vi "TLB Native Dynamic Events ver 0.07a.vi"() -> ()   [LabVIEW 2018]
uses:
  Labview Training Phase 2/Enum Controls/States for Action Engine.ctl
  Type def/TLB event states.ctl
  Type def/TLB MHL States.ctl
  <vilib>/Studica/Studica Toolkit/Background/I2C Channel.ctl
  <vilib>/Studica/Studica Toolkit/NavX/NavX.lvlib
  <vilib>/myRIO/Common/Instrument Driver Framework/myRIO v1.0/AI/typedefs/AI Channels Enum.ctl
  <vilib>/myRIO/Common/Instrument Driver Framework/myRIO v1.0/AI/typedefs/AI Channels List.ctl
  Type def/Type def.ctl
  Type def/Motor Control Cluster.ctl
  <vilib>/Studica/Studica Blackhawk/Blackhawk.lvlib
  <vilib>/userdefined/High Color/IMAQdx.ctl
  Underlying VI's/Webcam FGV Low level ver/State control.ctl
  <vilib>/Studica/Studica Toolkit/Background/Mxp Selection.ctl
  <vilib>/ptbypt/NI_PtbyPt.lvlib
  <vilib>/Studica/Studica Toolkit/Background/DIO Channel.ctl
  <vilib>/addons/control/pid/NI_PID_pid.lvlib
  <vilib>/addons/control/pid/pid.llb/PID (DBL).vi
  <vilib>/NI_Real-Time Target Support.lvlib
  <vilib>/Utility/RT CPU Load.ctl
panel:
  out "Load":errorcluster
  out "CPU loads":T1[](array[typedef]) {"ISR (%)" format="%#.2f"; "Idle (%)" format="%#.2f"; "Background (%)" format="%#.2f"; "Normal (%)" format="%#.2f"; "Above Normal (%)" format="%#.2f"; "High (%)" format="%#.2g"; "Timed Structures (%)" format="%#.2g"; "Time Critical (%)" format="%#.2g"; "Total (%)" format="%#.2g"}
  out "Waveform Chart":dbl(graph)
  in  "STOP":bool
  out "DIO 0":bool
  out "DIO 1":bool
  out "Limit Switch Array":bool[](array[boolean])
  out "Speed and distance cluster":T2
  out "error out":errorcluster
  out "Blackhawk loop":i32
  out "NavX Loop":i32
  out "Sensor Loop":i32
  out "User event loop":i32
  out "Event handling loop":i32
  out "Main Loop":i32
  out "Status loop":i32
  out "L/R average":fxp<+,64,64>
  out "Right Ultrasonic":fxp<+,64,16>
  out "Left Ultrasonic":fxp<+,64,16>
  out "Object detection count":T3
  out "Camera error":errorcluster
  out "Right IR Sensor":dbl
  out "Left IR Sensor":dbl
  in  "Servo Angle":u8(slide) scale=0.0..180.0
  in  "On/Off":bool
  out "Blackhawk error":errorcluster
  out "element":T4
  out "Action Queue Items":i32
  out "State Logic Queue Items":i32
  out "Action Queues items":string[](array[string])=["Hardware reset", "Software reset", ""]
  out "State logic":T5=enum."Task 2"
  out "Action State":string
  in  "Tasks Selector":string(combo)="Drive straight"
  out "Yaw":dbl
  out "NavX Info Out":T7
  out "LinearAcceleration":T8
  out "Displacement":T9
  out "YRPHfH":T10
  out "Object detected":bool
  in  "NavX Zero Yaw":bool
  # "Camera Status Loop"
  # "TLB FRAMEWORK STATUS"
  # "Test Programme written by Calvin Loke    Dated: 28 Aug 2019\nTest Programme revised by Dr Alex See   Dated 30 Aug 2019\n\nProgramme version:   TLB Native Dynamic Events ver 0.04b.vi"
  # "Sequence of Actions"
  # "Continuous (Repeated)"
  # "Motor Control Loop"
  # "Sensor data"
  # "Blackhawk status"
  # "System Health Status Update"
  # "NAVX Control Loop"
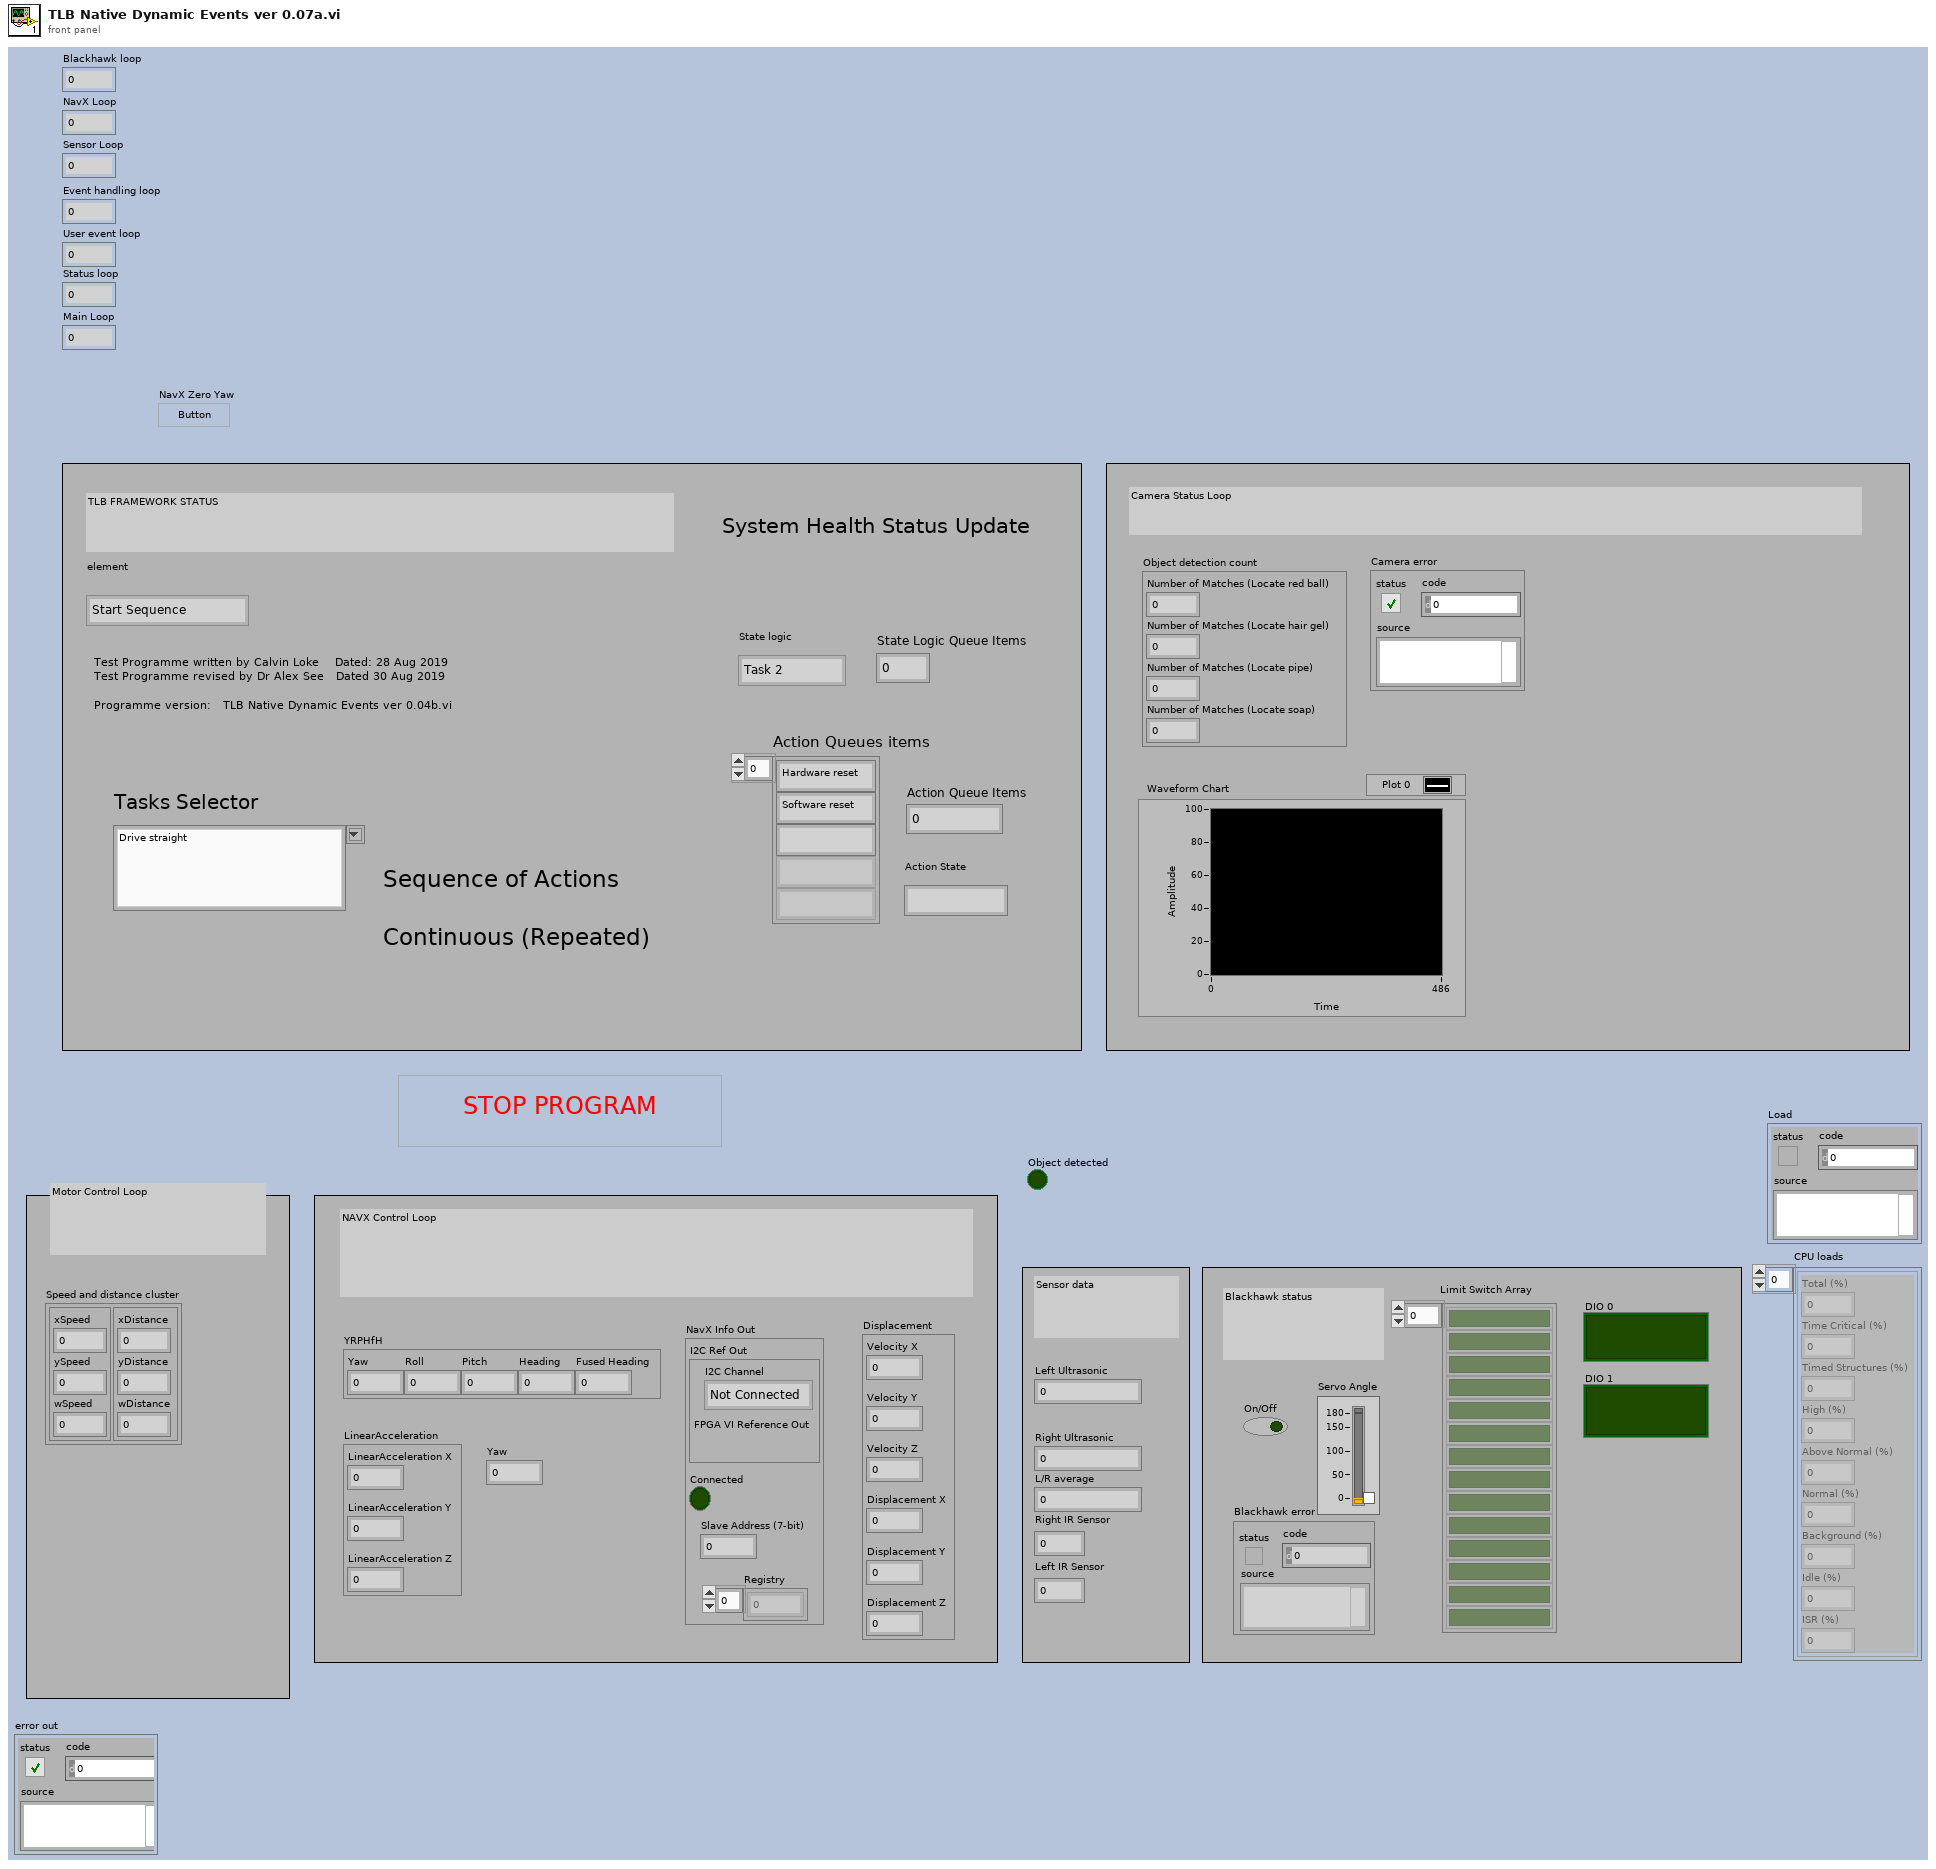
[diagram p1: front panel]
types:
  T1 = typedef "NI_Real-Time Target Support.lvlib/RT CPU Load.ctl" = cluster{"Total (%)":dbl, "Time Critical (%)":dbl, "Timed Structures (%)":dbl, "High (%)":dbl, "Above Normal (%)":dbl, "Normal (%)":dbl, "Background (%)":dbl, "Idle (%)":dbl, "ISR (%)":dbl}
  T2 = cluster{cluster{"xSpeed":dbl, "ySpeed":dbl, "wSpeed":dbl}, cluster{"xDistance":dbl, "yDistance":dbl, "wDistance":dbl}}
  T3 = cluster{"Number of Matches (Locate red ball)":i32, "Number of Matches (Locate hair gel)":i32, "Number of Matches (Locate pipe)":i32, "Number of Matches (Locate soap)":i32}
  T4 = typedef "TLB event states.ctl" = enum16{"Start Sequence", "Exit", "Start Task 1", "Start Task 2", "Start Task 3", "Start Task 4", "Camera vision", "Wall follow mode", "Idle", "Start Drive Straight"}
  T5 = typedef "TLB MHL States.ctl" = enum16{"None", "Startup", "Idle", "Processing", "Shutdown", "Reset", "Task 1", "Task 2", "Task 3", "Task 4", "Task 4a", "Task 4b", "Task 4c", "Task 4d", "Task 4e", "Task 4f", "Task 4g", "Task 4h", "Acquire image", "Wall follow mode", "Autodrive", "Autodrive a"}
  T6 = typedef "I2C Channel.ctl" = enum16{"Not Connected", "A", "B"}
  T7 = cluster{"I2C Ref Out":cluster{"I2C Channel":T6, "FPGA VI Reference Out":refnum<k20>}, "Connected":bool, "Slave Address (7-bit)":u8, "Registry":u8[]}
  T8 = cluster{"LinearAcceleration X":dbl, "LinearAcceleration Y":dbl, "LinearAcceleration Z":dbl}
  T9 = cluster{"Velocity X":dbl, "Velocity Y":dbl, "Velocity Z":dbl, "Displacement X":dbl, "Displacement Y":dbl, "Displacement Z":dbl}
  T10 = cluster{"Yaw":dbl, "Roll":dbl, "Pitch":dbl, "Heading":dbl, "Fused Heading":dbl}
  T11 = typedef "States for Action Engine.ctl" = enum16{"Initialize", "Write", "Read"}
  T12 = typedef "DIO Channel.ctl" = enum16{"Not Connected", "A/DIO1", "A/DIO2", "A/DIO3", "A/DIO4", "A/DIO5", "A/DIO6", "A/DIO7", "A/DIO13", "B/DIO1", "B/DIO2", "B/DIO3", "B/DIO4", "B/DIO5", "B/DIO6", "B/DIO7", "B/DIO13", "C/DIO0", "C/DIO1", "C/DIO2", "C/DIO3", "C/DIO4", "C/DIO5", "C/DIO6", "C/DIO7"}
  T13 = typedef "Motor Control Cluster.ctl" = cluster{"Vx":dbl, "Vy":dbl, "Vw":dbl}
  T14 = typedef "Type def.ctl" = cluster{"Front Ultrasonic Obstruct":bool, "Left Ultrasonic Obstruct":bool, "Right Ultrasonic Obstruct ":bool}
  T15 = typedef "Mxp Selection.ctl" = enum16{"MXP A", "MXP B"}
  T16 = typedef "TLB MHL States.ctl" = enum16{"None", "Startup", "Idle", "Processing", "Shutdown", "Reset", "Task 1", "Task 2", "Task 3", "Task 4", "Task 4a", "Task 4b", "Task 4c", "Task 4d", "Task 4e", "Task 4f", "Task 4g", "Task 4h", "Acquire image", "Wall follow mode", "Drive Straight"}
  T17 = cluster{"proportional gain (Kc)":dbl, "integral time (Ti, min)":dbl, "derivative time (Td, min)":dbl}
  T18 = typedef "State control.ctl" = enum16{"Initialise", "Start camera", "Continuous Acquisition ", "Stop camera", "Dispose all"}
  T19 = typedef "IMAQdx.ctl" = refnum<k21>
  T20 = cluster{"xTargetSpeed":dbl, "yTargetSpeed":dbl, "wTargetSpeed":dbl}
  T21 = cluster{"DIO Channel":T12, "FPGA VI Reference Out":refnum<k20>}
  T22 = typedef "IMAQ Image.ctl" = refnum<image>
  T23 = cluster{"xDistance":dbl, "yDistance":dbl, "wDistance":dbl}
  T24 = typedef "AI Channels List.ctl" = T25[]
  T25 = typedef "AI Channels Enum.ctl" = enum16{"Not Connected", "AudioIn/Left", "AudioIn/Right", "C/AI0", "C/AI1", "A/AI0", "A/AI1", "A/AI2", "A/AI3", "A/AI4", "A/AI5", "A/AI6", "A/AI7", "B/AI0", "B/AI1", "B/AI2", "B/AI3", "B/AI4", "B/AI5", "B/AI6", "B/AI7", "AI/AI0", "AI/AI1", "AI/AI2", "AI/AI3", "A/AI0 (DIFF)", "A/AI1 (DIFF)", "A/AI2 (DIFF)", "A/AI3 (DIFF)", "B/AI0 (DIFF)", "B/AI1 (DIFF)", "B/AI2 (DIFF)", "B/AI3 (DIFF)"}
  T26 = cluster{"I2C Channel":T6, "FPGA VI Reference Out":refnum<k20>}
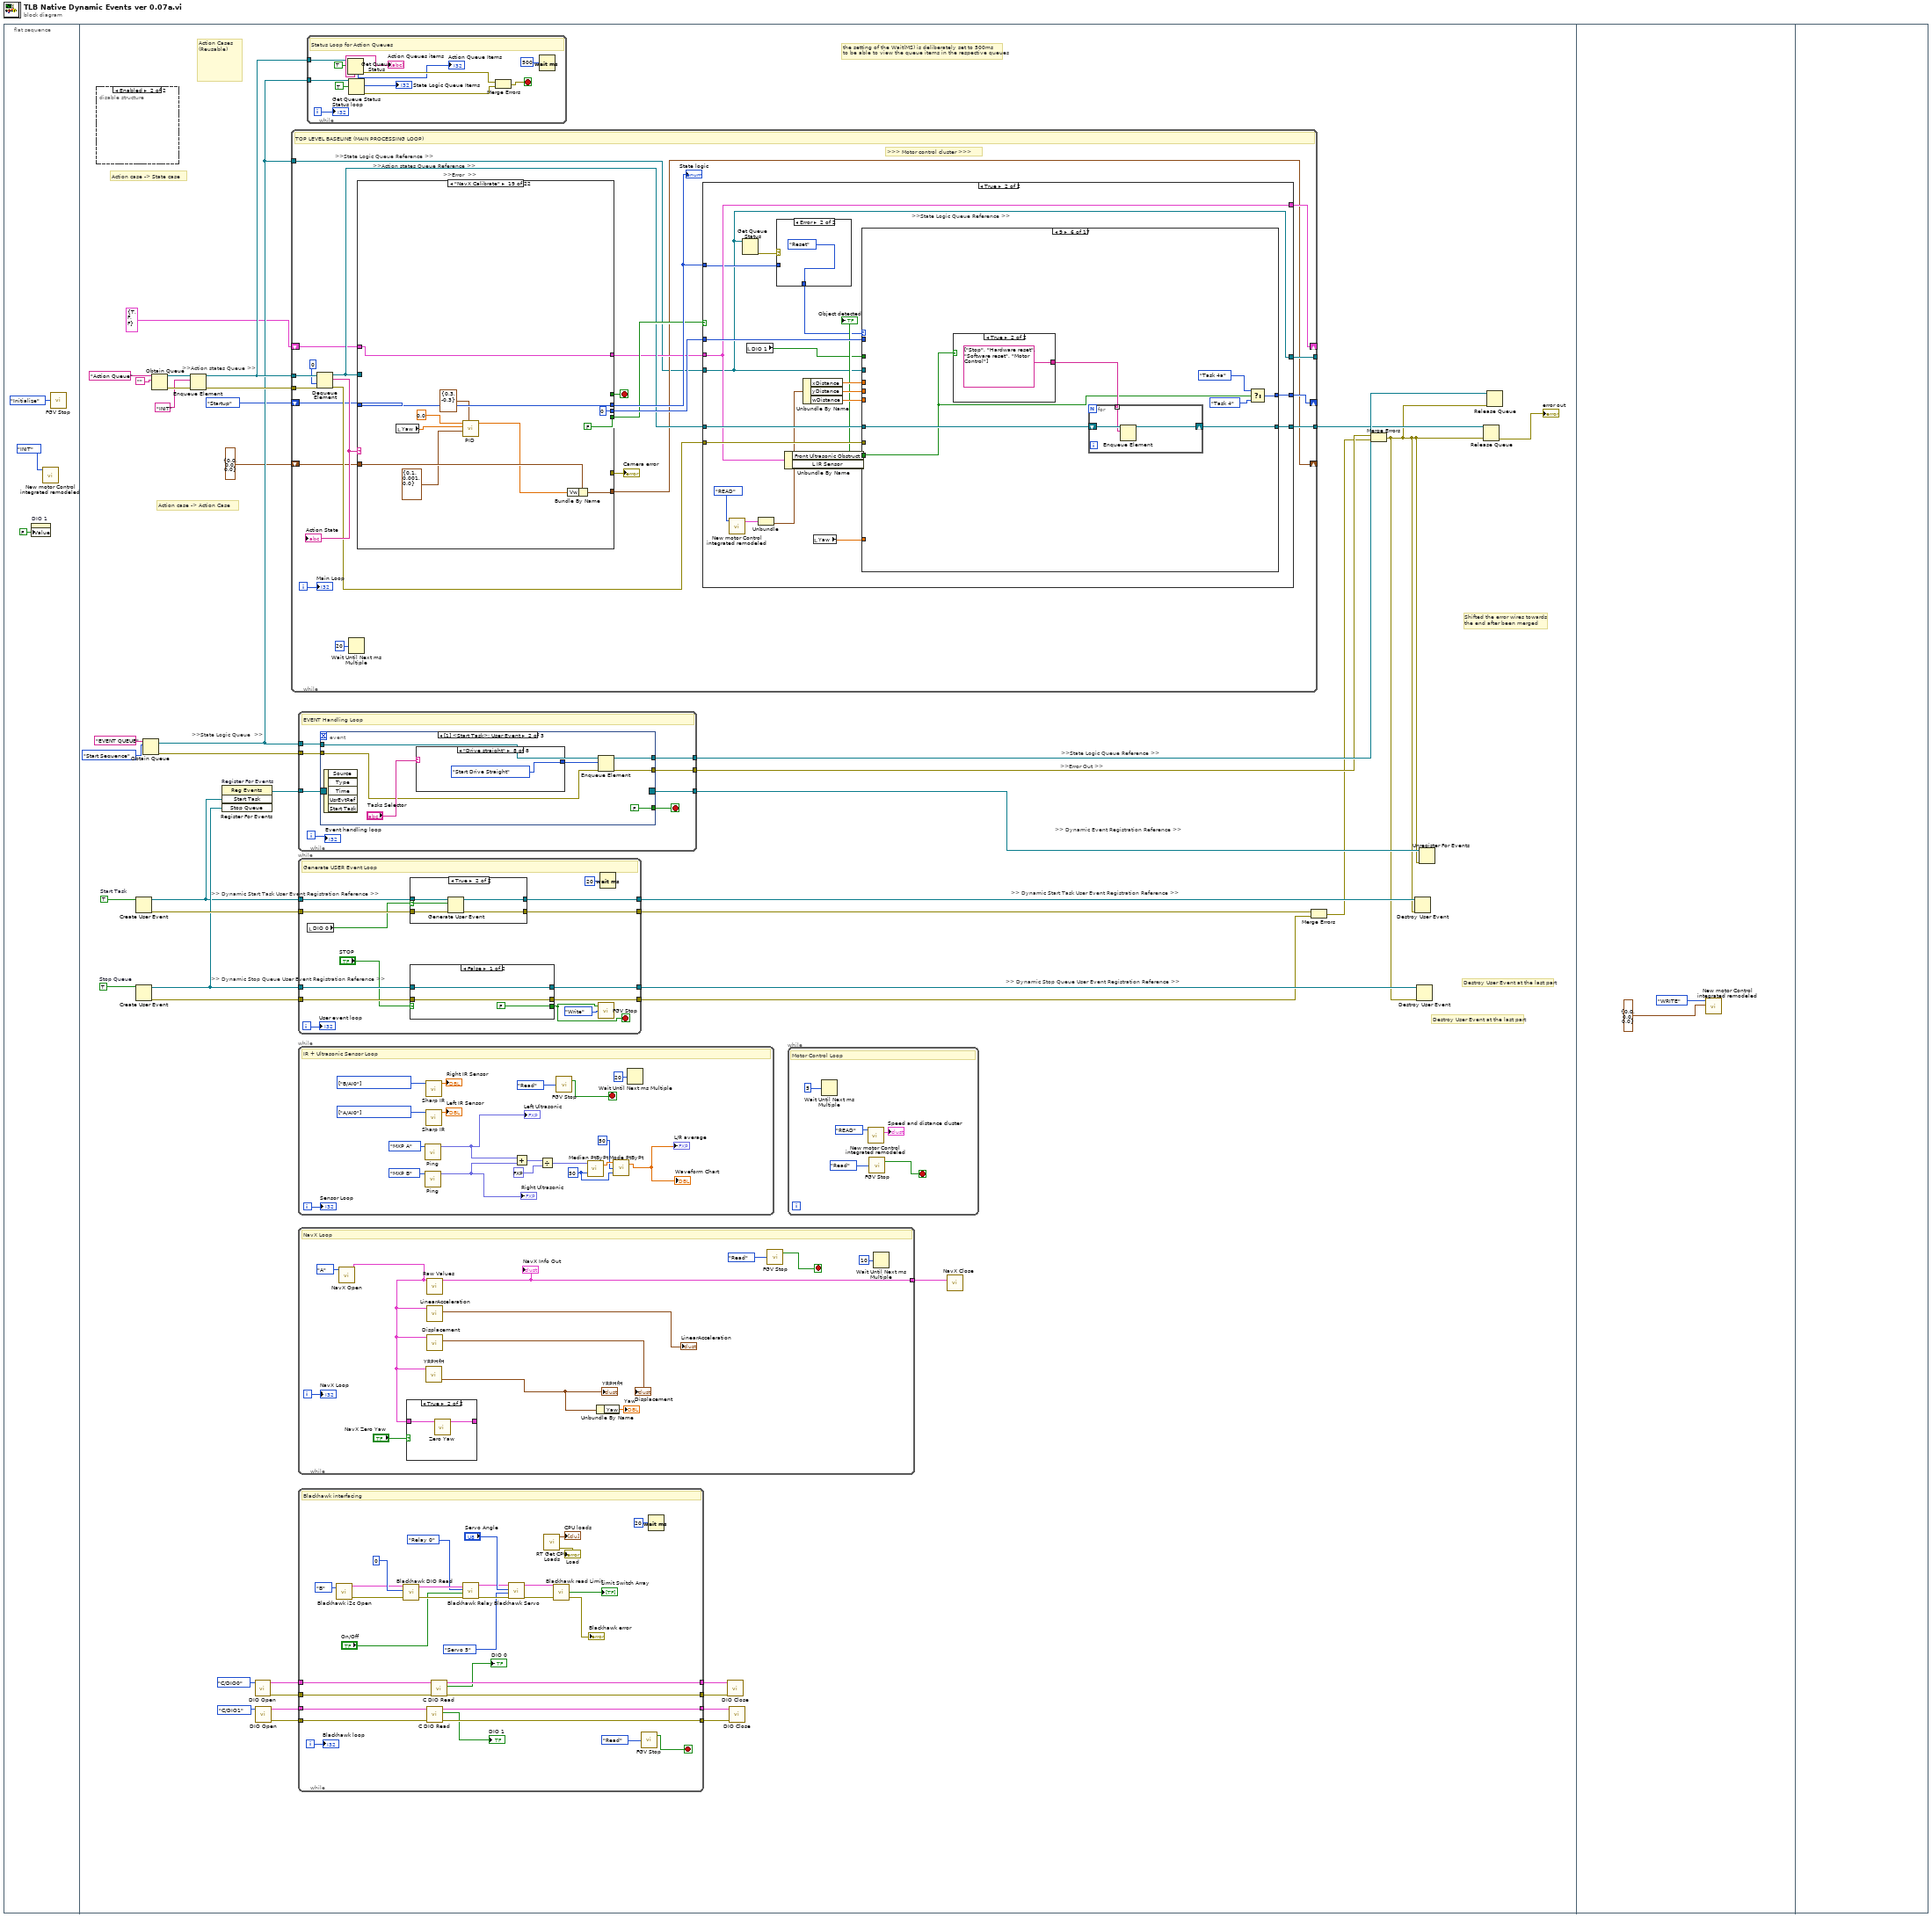
[diagram p0: block diagram]
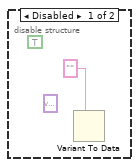
[diagram p3: hidden frame]
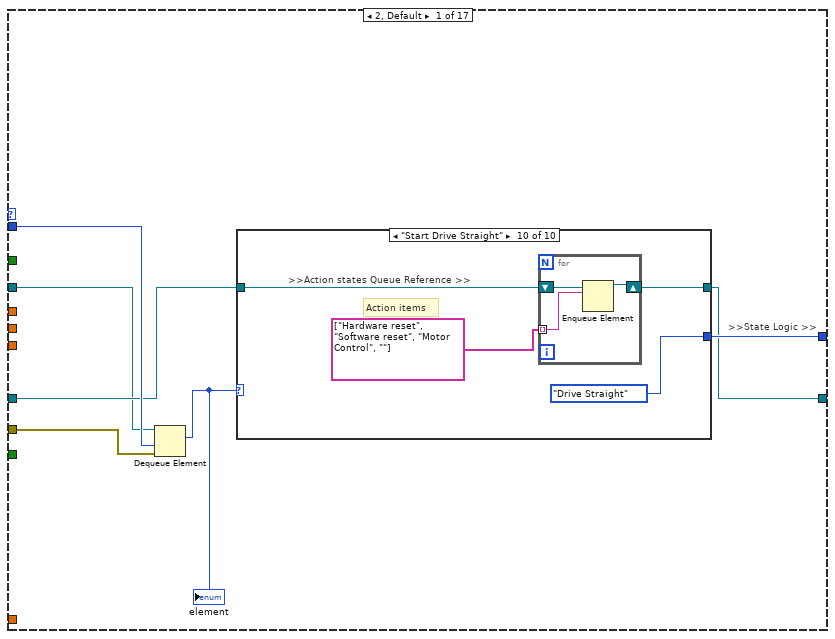
[diagram p6: hidden frame]
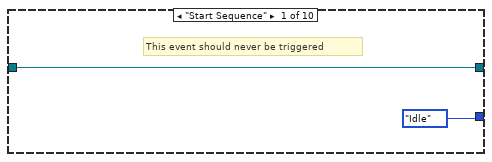
[diagram p7: hidden frame]
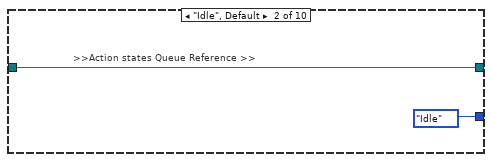
[diagram p8: hidden frame]
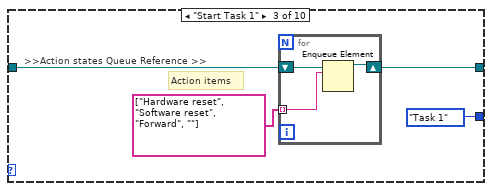
[diagram p9: hidden frame]
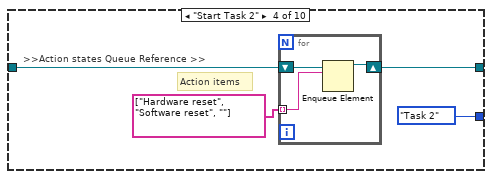
[diagram p10: hidden frame]
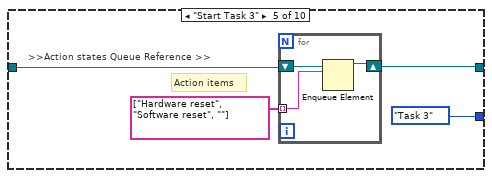
[diagram p11: hidden frame]
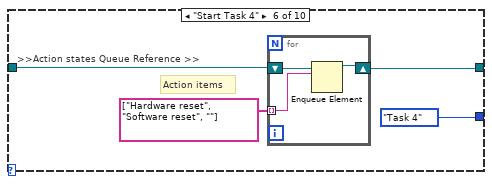
[diagram p12: hidden frame]
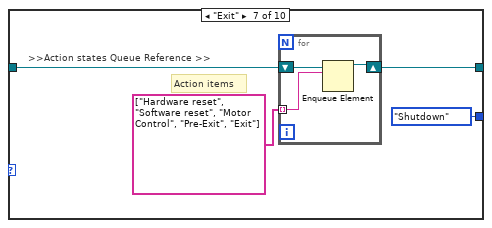
[diagram p13: hidden frame]
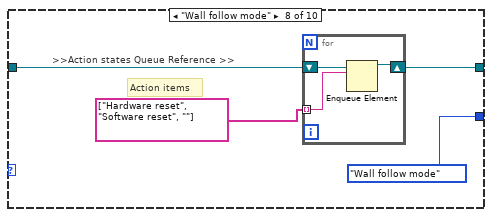
[diagram p14: hidden frame]
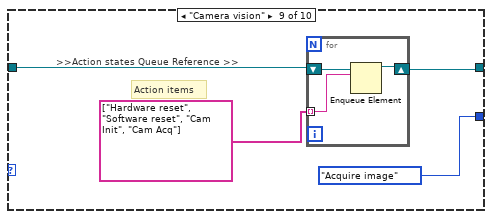
[diagram p15: hidden frame]
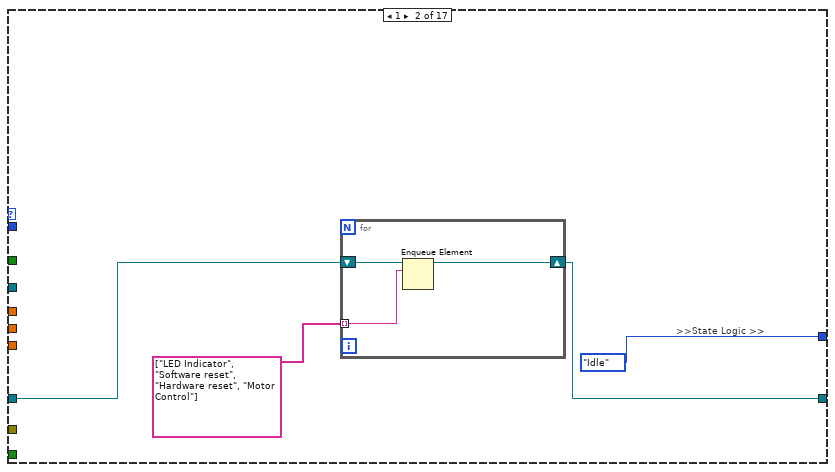
[diagram p16: hidden frame]
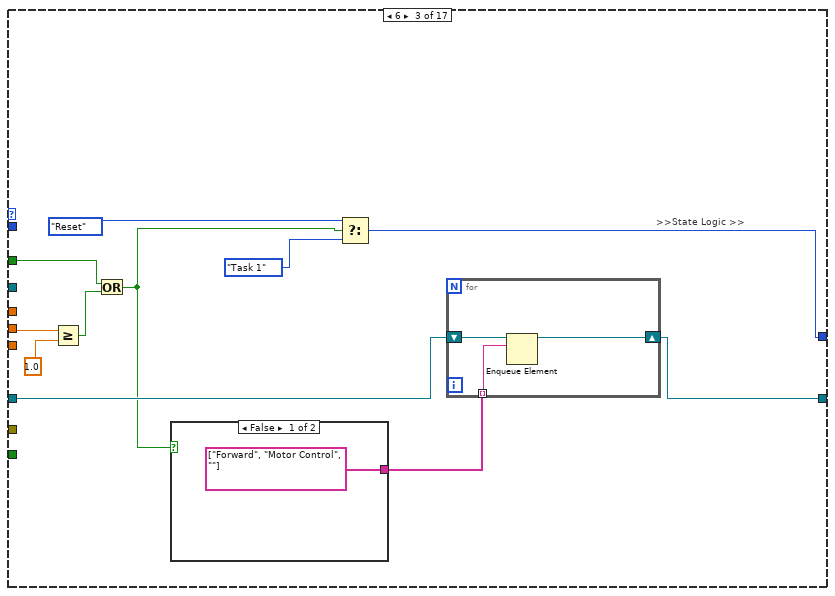
[diagram p17: hidden frame]
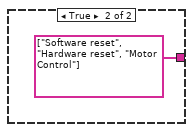
[diagram p18: hidden frame]
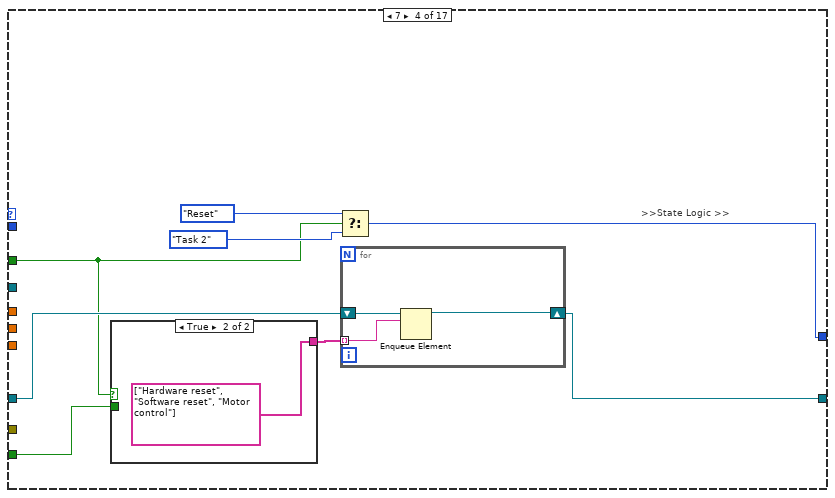
[diagram p19: hidden frame]
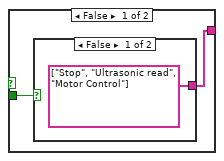
[diagram p20: hidden frame]
diagram:
  n1 = flat-sequence {
    frame #0 {
      n2 = property on="DIO 1" class="Bool (strict)"("Value"=FALSE ("DIO 1")) -> ()  [unwired: 2 in, 2 out]
      n3 = call "New motor Control integrated remodeled.vi"("States"=enum16{"RESET ENCODER", "WRITE", "READ", "INIT"}."INIT") -> ()  [unwired: 4 in, 2 out]
      n4 = call "FGV Stop.vi"("Init/Read/Write State"=States_for_Action_Engine."Initialize") -> ()  [unwired: 2 in, 2 out]
    }
    frame #1 {
      w46 = TRUE  # Stop Queue
      w45 = TRUE  # Start Task
      # "Action case -> Action Case"
      # "Action case -> State case"
      # "the setting of the Wait(MS) is deliberately set to 500ms\nto be able to view the queue items in the respective queues"
      # "Action Cases\n(Reusable)"
      # ">>Error Out >>"
      # ">> Dynamic Stop Queue User Event Registration Reference >>"
      # ">> Dynamic Start Task User Event Registration Reference >>"
      # ">> Dynamic Stop Queue User Event Registration Reference >>"
      # ">> Dynamic Start Task User Event Registration Reference >>"
      # ">> Dynamic Event Registration Reference >>"
      # ">>Action states Queue >>"
      # ">>State Logic Queue  >>"
      # ">>State Logic Queue Reference >>"
      # "Destroy User Event at the last part"
      # "Destroy User Event at the last part"
      # "Shifted the error wires towards\nthe end after been merged"
      n5 = disable-structure shown="Enabled" {
        frame Disabled {
          (unwired) variant
          (unwired) TRUE
          n6 = Variant To Data(type="") -> ()  [unwired: 2 in, 2 out]
        }
        frame Enabled {
        }
      }
      n7 = Create User Event(user event datatype=w45) -> (user event=w37:refnum<user-event>, error out=w42:errorcluster)  [unwired: 1 in]
      n8 = Create User Event(user event datatype=w46) -> (user event=w38:refnum<user-event>, error out=w41:errorcluster)  [unwired: 1 in]
      n9 = Obtain Queue(name (unnamed)="EVENT QUEUE", element data type=TLB_event_states."Start Sequence" ("Enum")) -> (queue out=w22:refnum<queue>, error out=w28:errorcluster)  [unwired: 3 in, 1 out]
      n10 = Obtain Queue(name (unnamed)="Action Queue", element data type="") -> (queue out=w31:refnum<queue>, error out=w27:errorcluster)  [unwired: 3 in, 1 out]
      n11 = Enqueue Element(queue=w31, element="INIT", error in (no error)=w27) -> (queue out=w23:refnum<queue>, error out=w26:errorcluster)  [unwired: 1 in, 1 out]
      n12 = register-events "Register For Events"(w37, w38) -> (reference out=w36:refnum<event-registration>)  [unwired: 2 in, 1 out]
      n13 = call <vilib>:"DIO Open.vi"("DIO Channel"=DIO_Channel."C/DIO0") -> ("error out"=w10:errorcluster, "DIO Info Out"=w16:T21)  [unwired: 9 in]
      n14 = call <vilib>:"DIO Open.vi"("DIO Channel"=DIO_Channel."C/DIO1") -> ("error out"=w8:errorcluster, "DIO Info Out"=w12:T21)  [unwired: 9 in]
      n15 = while {
        tunnel: w22 -> [w133]
        shift-right: [w147] -> _
        shift-left: TLB_MHL_States."Startup" ("Enum") -> [w141]
        tunnel: w23 -> [w152]
        tunnel: w26 -> [w150]
        tunnel: [w149] -> _
        tunnel: [w148] -> w6
        shift-right: [w138] -> _
        shift-left: T14 {"Front Ultrasonic Obstruct"=TRUE, "Left Ultrasonic Obstruct"=FALSE, "Right Ultrasonic Obstruct "=FALSE} -> [w140]
        shift-right: [w136] -> _
        shift-left: T13 {"Vx"=0.0, "Vy"=0.0, "Vw"=0.0} -> [w137]
        i -> [w134]
        stop <- w131 stop-if-true
        # ">>> Motor control cluster >>>"
        # ">>Error  >>"
        # ">>Action states Queue Reference >>"
        # ">>State Logic Queue Reference >>"
        # "TOP LEVEL BASELINE (MAIN PROCESSING LOOP)"
        n16 = Dequeue Element(queue=w152, timeout in ms (-1)=0, error in (no error)=w150) -> (queue out=w142:refnum<queue>, element=w151:string, error out=w143:errorcluster)  [unwired: 1 out]
        "Action State" <- w151
        n17 = Wait Until Next ms Multiple(millisecond multiple=u32 20) -> ()  [unwired: 1 out]
        n18 = case shown="\"NavX Calibrate\"" w151 {
          tunnel: [w428 w440 w445 w452 w460 w469 w477 w483 w493 w500 w506 w516 w526 TLB_MHL_States."Shutdown" ("Enum") w537 w547 w551 w566 w576 w589 w597 w611] -> w153
          tunnel: [w432 0 0 0 0 0 0 0 0 0 0 0 0 0 0 0 0 0 0 0 0 0] -> w146
          tunnel: [TRUE FALSE FALSE FALSE FALSE FALSE FALSE FALSE FALSE FALSE FALSE FALSE FALSE FALSE FALSE FALSE FALSE FALSE FALSE FALSE FALSE FALSE] -> w145
          tunnel: w142 -> [_ _ _ _ _ _ _ _ _ _ _ _ _ _ _ _ _ _ _ _ _ _]
          tunnel: w141 -> [w428 w440 w445 w452 w460 w469 w477 w483 w493 w500 w506 w516 w526 _ w537 w547 w551 w566 w576 w589 w597 w611]
          tunnel: w140 -> [w430 w437 w442 w449 w457 w465 w473 w481 w489 w497 w507 w513 w522 w529 w538 w546 w554 w567 w574 w590 w596 w607]
          tunnel: [w430 w437 w442 w449 w457 w465 w473 w481 w489 w497 w507 w512 w522 w529 w538 w543 w553 w567 w574 w590 w596 w607] -> w139
          tunnel: w137 -> [w429 w436 w441 w447 w455 w463 w472 w479 w488 w495 w503 w510 w521 w528 w534 w540 w548 w562 w577 w588 w600 w608]
          tunnel: [w429 w436 w441 w448 w456 w464 w471 w480 w487 w496 w503 w510 w519 w528 w534 w540 w548 w563 w578 w588 w600 w608] -> w136
          tunnel: [_ _ _ _ _ _ _ _ _ _ _ _ _ _ _ _ _ _ _ w579 w592 w601] -> w135
          tunnel: [_ _ _ _ _ _ _ _ _ _ _ _ _ TRUE _ _ _ _ _ _ _ _] -> w131
          frame "No action", Default {
            n19 = case shown="1, Default" w428 {
              tunnel: [0 100] -> w432
              frame 1, Default {
              }
              frame 2 {
              }
            }
          }
          frame "Init" {
            # ">>State Logic  >>"
            n20 = local write "Servo Angle"(u8 90 ("Servo Angle")) -> ()
          }
          frame "LED Indicator" {
          }
          frame "Forward" {
            n21 = local write "NavX Zero Yaw"(FALSE ("NavX Zero Yaw")) -> ()
            n22 = Bundle By Name(cluster=w447, "Vy"=0.6) -> (w448:T13)
          }
          frame "Reverse" {
            n23 = local write "NavX Zero Yaw"(FALSE ("NavX Zero Yaw")) -> ()
            n24 = Bundle By Name(cluster=w455, "Vy"=-0.6) -> (w456:T13)
          }
          frame "Right" {
            n25 = local write "NavX Zero Yaw"(FALSE ("NavX Zero Yaw")) -> ()
            n26 = Bundle By Name(cluster=w463, "Vx"=0.6) -> (w464:T13)
          }
          frame "Left" {
            n27 = Bundle By Name(cluster=w472, "Vx"=-0.6) -> (w471:T13)
            n28 = local write "NavX Zero Yaw"(FALSE ("NavX Zero Yaw")) -> ()
          }
          frame "Rotate CW" {
            n29 = local write "NavX Zero Yaw"(FALSE ("NavX Zero Yaw")) -> ()
            n30 = Bundle By Name(cluster=w479, "Vw"=-0.3) -> (w480:T13)
          }
          frame "Rotate ACW" {
            n31 = local write "NavX Zero Yaw"(FALSE ("NavX Zero Yaw")) -> ()
            n32 = Bundle By Name(cluster=w488, "Vw"=0.15) -> (w487:T13)
          }
          frame "Stop" {
            w494 = 0.0
            n33 = local write "NavX Zero Yaw"(FALSE ("NavX Zero Yaw")) -> ()
            n34 = Bundle By Name(cluster=w495, "Vx"=w494, "Vy"=w494, "Vw"=w494) -> (w496:T13)
          }
          frame "Motor control" {
            n35 = call "New motor Control integrated remodeled.vi"("States"=enum16{"RESET ENCODER", "WRITE", "READ", "INIT"}."WRITE", "Target Speed"=w503) -> ()  [unwired: 3 in, 2 out]
          }
          frame "Software reset" {
            w511 = FALSE ("NavX Zero Yaw")
            n36 = Wait (ms)(milliseconds to wait=u32 20) -> ()  [unwired: 1 out]
            n37 = local write "NavX Zero Yaw"(w511) -> ()
            n38 = Bundle By Name(cluster=w513, "Front Ultrasonic Obstruct"=w511, "L IR Sensor"=0.0) -> (w512:T14)
          }
          frame "Hardware reset" {
            w520 = 0.0
            n39 = Wait (ms)(milliseconds to wait=u32 20) -> ()  [unwired: 1 out]
            n40 = local write "NavX Zero Yaw"(TRUE ("NavX Zero Yaw")) -> ()
            n41 = call "New motor Control integrated remodeled.vi"("States"=enum16{"RESET ENCODER", "WRITE", "READ", "INIT"}."RESET ENCODER") -> ()  [unwired: 4 in, 2 out]
            n42 = Bundle By Name(cluster=w521, "Vx"=w520, "Vy"=w520, "Vw"=w520) -> (w519:T13)
          }
          frame "Exit" {
          }
          frame "Pre-Exit" {
            n43 = call "New motor Control integrated remodeled.vi"("States"=enum16{"RESET ENCODER", "WRITE", "READ", "INIT"}."INIT") -> ()  [unwired: 4 in, 2 out]
          }
          frame "Ultrasonic read" {
            # "Object detection"
            n44 = local read "L/R average"() -> (w539:fxp<+,64,64>)
            n45 = Less Or Equal?(x=w539, y=35.0) -> (x <= y?=w541:bool)
            n46 = Bundle By Name(cluster=w546, "Front Ultrasonic Obstruct"=w541) -> (w543:T14)
          }
          frame "IR Sensor Read" {
            n47 = local read "Left IR Sensor"() -> (w552:dbl)
            n48 = Bundle By Name(cluster=w554, "L IR Sensor"=w552) -> (w553:T14)
          }
          frame "Calculate" {
            n49 = Unbundle By Name(w567) -> ("L IR Sensor"=w559:dbl)
            n50 = call-poly <vilib>:"PID.vi"("output range"=cluster{"output high":dbl, "output low":dbl} {"output high"=0.3, "output low"=-0.3}, "PID gains"=T17 {"proportional gain (Kc)"=0.01, "integral time (Ti, min)"=0.0, "derivative time (Td, min)"=0.0}, "process variable"=w559, "setpoint"=20.0) -> ("output"=w556:dbl)  [unwired: 6 in, 1 out]
            n51 = Negate(x=w556) -> (-x=w555:dbl)
            n52 = Bundle By Name(cluster=w562, "Vy"=0.2, "Vw"=w555) -> (w563:T13)
          }
          frame "NavX Calibrate" {
            n53 = local read "Yaw"() -> (w571:dbl)
            n54 = call-poly <vilib>:"PID.vi"("output range"=cluster{"output high":dbl, "output low":dbl} {"output high"=0.3, "output low"=-0.3}, "PID gains"=T17 {"proportional gain (Kc)"=0.1, "integral time (Ti, min)"=0.001, "derivative time (Td, min)"=0.0}, "process variable"=w571, "setpoint"=0.0 ("y")) -> ("output"=w568:dbl)  [unwired: 6 in, 1 out]
            n55 = Bundle By Name(cluster=w577, "Vw"=w568) -> (w578:T13)
          }
          frame "Cam Init" {
            n56 = call "Low-Level Grab.vi"("States"=State_control."Initialise", "Session In"=T19 "cam1") -> ("error out"=w580:errorcluster, "Session Out"=w581:T19)  [unwired: 7 in, 1 out]
            n57 = call "Low-Level Grab.vi"("error in (no error)"=w580, "States"=State_control."Start camera", "Session In"=w581) -> ("error out"=w579:errorcluster)  [unwired: 6 in, 2 out]
            n58 = local write "Servo Angle"(u8 170 ("Servo Angle")) -> ()
          }
          frame "Cam Acq" {
            n59 = call "Low-Level Grab.vi"("States"=State_control."Continuous Acquisition ") -> ("error out"=w593:errorcluster, "Image Out"=w594:T22)  [unwired: 8 in, 1 out]
            n60 = call "All object detection ver2.vi"("Image In"=w594, "error in"=w593) -> ("Object detection count"=→"Object detection count":T3, "error out"=w592:errorcluster)  [unwired: 1 out]
          }
          frame "Cam Exit" {
            n61 = call "Low-Level Grab.vi"("States"=State_control."Stop camera") -> ("error out"=w602:errorcluster, "Session Out"=w604:T19)  [unwired: 8 in, 1 out]
            n62 = local write "Servo Angle"(u8 90 ("Servo Angle")) -> ()
            n63 = call "Low-Level Grab.vi"("error in (no error)"=w602, "States"=State_control."Dispose all", "Session In"=w604) -> ("error out"=w601:errorcluster)  [unwired: 6 in, 2 out]
          }
        }
        "State logic" <- w153
        "Camera error" <- w135
        n64 = case shown="True" w145 {
          tunnel: w153 -> [w156 w161]
          tunnel: w133 -> [w157 w160]
          tunnel: w142 -> [w155 w176]
          tunnel: [w157 w160] -> w149
          tunnel: [w155 w175] -> w148
          tunnel: [w156 w174] -> w147
          tunnel: w143 -> [_ w173]
          tunnel: w146 -> [_ w172]
          tunnel: w139 -> [w154 w166]
          tunnel: [w154 w166] -> w138
          frame False {
          }
          frame True {
            # ">>State Logic Queue Reference >>"
            n65 = call "New motor Control integrated remodeled.vi"("States"=enum16{"RESET ENCODER", "WRITE", "READ", "INIT"}."READ") -> ("Speed and distance cluster"=w165:T2)  [unwired: 4 in, 1 out]
            n66 = Get Queue Status(queue=w160) -> (error out=w159:errorcluster)  [unwired: 2 in, 7 out]
            n67 = local read "DIO 1"() -> (w158:bool)
            n68 = Unbundle(w165) -> (w164:T23)  [unwired: 1 out]
            n69 = case shown="Error" w159 {
              tunnel: [w177 TLB_MHL_States."Reset" ("Enum")] -> w162
              tunnel: w161 -> [w177 _]
              frame No Error {
              }
              frame Error {
              }
            }
            n70 = Unbundle By Name(w166) -> ("Front Ultrasonic Obstruct"=w167:bool)  [unwired: 1 out]
            "Object detected" <- w167
            n71 = Unbundle By Name(w164) -> ("xDistance"=w169:dbl, "yDistance"=w171:dbl, "wDistance"=w170:dbl)
            n72 = local read "Yaw"() -> (w168:dbl)
            n73 = case shown="9" w162 {
              tunnel: w160 -> [w179 _ _ _ _ _ _ _ _ _ _ _ _ _ _ _ _]
              tunnel: w176 -> [w181 w247 w259 w272 w294 w303 w317 w332 w345 w360 w370 w378 w394 w408 w417 w420 w426]
              tunnel: [w180 w246 w258 w273 w293 w304 w316 w331 w344 w359 w369 w379 w395 w407 w417 w419 w426] -> w175
              tunnel: [w184 TLB_MHL_States."Idle" ("Enum") w261 w274 w290 w307 w319 w330 w346 w358 TLB_MHL_States."Shutdown" ("Enum") w381 w396 w406 TLB_MHL_States."Reset" ("Enum") TLB_MHL_States."Shutdown" ("Enum") TLB_MHL_States."Reset" ("Enum")] -> w174
              tunnel: w173 -> [w182 _ _ _ _ _ _ _ _ _ _ _ _ _ _ _ _]
              tunnel: w172 -> [w183 _ _ _ _ _ _ _ _ _ _ _ _ _ _ _ _]
              tunnel: w158 -> [_ _ w256 w271 w288 _ _ _ _ w357 _ w376 w392 w405 _ _ _]
              tunnel: w171 -> [_ _ w253 _ _ _ _ w327 _ _ _ _ _ _ _ _ _]
              tunnel: w170 -> [_ _ _ _ w285 _ _ _ _ _ _ _ _ _ _ _ _]
              tunnel: w169 -> [_ _ _ _ _ _ w313 _ w341 _ _ _ _ _ _ _ _]
              tunnel: w168 -> [_ _ _ _ _ _ _ _ _ _ _ _ _ _ _ _ _]
              tunnel: w167 -> [_ _ _ w269 _ w301 _ _ _ w356 _ _ w389 _ _ _ _]
              frame 2, Default {
                # ">>State Logic >>"
                n74 = Dequeue Element(queue=w179, timeout in ms (-1)=w183, error in (no error)=w182) -> (element=w185:T4)  [unwired: 3 out]
                "element" <- w185
                n75 = case shown="\"Start Drive Straight\"" w185 {
                  tunnel: [TLB_MHL_States."Idle" ("Enum") TLB_MHL_States."Idle" ("Enum") TLB_MHL_States."Task 1" ("Enum") TLB_MHL_States."Task 2" ("Enum") TLB_MHL_States."Task 3" ("Enum") TLB_MHL_States."Task 4" ("Enum") TLB_MHL_States."Shutdown" ("Enum") TLB_MHL_States."Wall follow mode" ("Enum") TLB_MHL_States."Acquire image" ("Enum") TLB_MHL_States."Drive Straight" ("Enum")] -> w184
                  tunnel: [w187 w188 w192 w197 w206 w212 w218 w225 w233 w240] -> w180
                  tunnel: w181 -> [w187 w188 w190 w198 w207 w213 w219 w226 w234 w241]
                  frame "Start Sequence" {
                    # "This event should never be triggered"
                  }
                  frame "Idle", Default {
                    # ">>Action states Queue Reference >>"
                  }
                  frame "Start Task 1" {
                    # ">>Action states Queue Reference >>"
                    # "Action items"
                    n76 = for {
                      shift-right: [w196] -> w192
                      shift-left: w190 -> [w195]
                      tunnel: string[] ["Hardware reset", "Software reset", "Forward", ""] -> [w194] mode=indexing
                      n77 = Enqueue Element(queue=w195, element=w194) -> (queue out=w196:refnum<queue>)  [unwired: 2 in, 2 out]
                    }
                  }
                  frame "Start Task 2" {
                    # ">>Action states Queue Reference >>"
                    # "Action items"
                    n78 = for {
                      shift-right: [w203] -> w197
                      shift-left: w198 -> [w202]
                      tunnel: string[] ["Hardware reset", "Software reset", ""] -> [w201] mode=indexing
                      n79 = Enqueue Element(queue=w202, element=w201) -> (queue out=w203:refnum<queue>)  [unwired: 2 in, 2 out]
                    }
                  }
                  frame "Start Task 3" {
                    # ">>Action states Queue Reference >>"
                    # "Action items"
                    n80 = for {
                      shift-right: [w210] -> w206
                      shift-left: w207 -> [w209]
                      tunnel: string[] ["Hardware reset", "Software reset", ""] -> [w208] mode=indexing
                      n81 = Enqueue Element(queue=w209, element=w208) -> (queue out=w210:refnum<queue>)  [unwired: 2 in, 2 out]
                    }
                  }
                  frame "Start Task 4" {
                    # ">>Action states Queue Reference >>"
                    # "Action items"
                    n82 = for {
                      shift-right: [w217] -> w212
                      shift-left: w213 -> [w216]
                      tunnel: string[] ["Hardware reset", "Software reset", ""] -> [w215] mode=indexing
                      n83 = Enqueue Element(queue=w216, element=w215) -> (queue out=w217:refnum<queue>)  [unwired: 2 in, 2 out]
                    }
                  }
                  frame "Exit" {
                    # ">>Action states Queue Reference >>"
                    # "Action items"
                    n84 = for {
                      shift-right: [w224] -> w218
                      shift-left: w219 -> [w223]
                      tunnel: string[] ["Hardware reset", "Software reset", "Motor Control", "Pre-Exit", "Exit"] -> [w222] mode=indexing
                      n85 = Enqueue Element(queue=w223, element=w222) -> (queue out=w224:refnum<queue>)  [unwired: 2 in, 2 out]
                    }
                  }
                  frame "Wall follow mode" {
                    # ">>Action states Queue Reference >>"
                    # "Action items"
                    n86 = for {
                      shift-right: [w231] -> w225
                      shift-left: w226 -> [w230]
                      tunnel: string[] ["Hardware reset", "Software reset", ""] -> [w229] mode=indexing
                      n87 = Enqueue Element(queue=w230, element=w229) -> (queue out=w231:refnum<queue>)  [unwired: 2 in, 2 out]
                    }
                  }
                  frame "Camera vision" {
                    # ">>Action states Queue Reference >>"
                    # "Action items"
                    n88 = for {
                      shift-right: [w238] -> w233
                      shift-left: w234 -> [w237]
                      tunnel: string[] ["Hardware reset", "Software reset", "Cam Init", "Cam Acq"] -> [w236] mode=indexing
                      n89 = Enqueue Element(queue=w237, element=w236) -> (queue out=w238:refnum<queue>)  [unwired: 2 in, 2 out]
                    }
                  }
                  frame "Start Drive Straight" {
                    # ">>Action states Queue Reference >>"
                    # "Action items"
                    n90 = for {
                      shift-right: [w245] -> w240
                      shift-left: w241 -> [w244]
                      tunnel: string[] ["Hardware reset", "Software reset", "Motor Control", ""] -> [w243] mode=indexing
                      n91 = Enqueue Element(queue=w244, element=w243) -> (queue out=w245:refnum<queue>)  [unwired: 2 in, 2 out]
                    }
                  }
                }
              }
              frame 1 {
                # ">>State Logic >>"
                n92 = for {
                  shift-right: [w251] -> w246
                  shift-left: w247 -> [w252]
                  tunnel: string[] ["LED Indicator", "Software reset", "Hardware reset", "Motor Control"] -> [w250] mode=indexing
                  n93 = Enqueue Element(queue=w252, element=w250) -> (queue out=w251:refnum<queue>)  [unwired: 2 in, 2 out]
                }
              }
              frame 6 {
                # ">>State Logic >>"
                n94 = Greater Or Equal?(x=w253, y=1.0) -> (x >= y?=w254:bool)
                n95 = Or(x=w256, y=w254) -> (x .or. y?=w257:bool)
                n96 = case shown="False" w257 {
                  tunnel: [string[] ["Forward", "Motor Control", ""] string[] ["Software reset", "Hardware reset", "Motor Control"]] -> w260
                  frame False {
                  }
                  frame True {
                  }
                }
                n97 = Select(t=TLB_MHL_States."Reset" ("Enum"), s=w257, f=TLB_MHL_States."Task 1" ("Enum")) -> (s? t:f=w261:T5)
                n98 = for {
                  shift-right: [w267] -> w258
                  shift-left: w259 -> [w268]
                  tunnel: w260 -> [w266] mode=indexing
                  n99 = Enqueue Element(queue=w268, element=w266) -> (queue out=w267:refnum<queue>)  [unwired: 2 in, 2 out]
                }
              }
              frame 7 {
                # ">>State Logic >>"
                n100 = case shown="True" w271 {
                  tunnel: [w278 string[] ["Hardware reset", "Software reset", "Motor control"]] -> w270
                  tunnel: w269 -> [w277 _]
                  frame False {
                    n101 = case shown="False" w277 {
                      tunnel: [string[] ["Stop", "Ultrasonic read", "Motor Control"] string[] ["Reverse", "Ultrasonic read", "Motor control"]] -> w278
                      frame False {
                      }
                      frame True {
                      }
                    }
                  }
                  frame True {
                  }
                }
                n102 = Select(t=TLB_MHL_States."Reset" ("Enum"), s=w271, f=TLB_MHL_States."Task 2" ("Enum")) -> (s? t:f=w274:T5)
                n103 = for {
                  shift-right: [w283] -> w273
                  shift-left: w272 -> [w284]
                  tunnel: w270 -> [w282] mode=indexing
                  n104 = Enqueue Element(queue=w284, element=w282) -> (queue out=w283:refnum<queue>)  [unwired: 2 in, 2 out]
                }
              }
              frame 8 {
                n105 = Less Or Equal?(x=w285, y=-1.2) -> (x <= y?=w286:bool)
                n106 = Or(x=w286, y=w288) -> (x .or. y?=w289:bool)
                n107 = case shown="True" w289 {
                  tunnel: [string[] ["Rotate CW", "Motor Control"] string[] ["Software reset", "Hardware reset", "Motor Control"]] -> w295
                  frame False {
                  }
                  frame True {
                  }
                }
                n108 = for {
                  shift-right: [w297] -> w293
                  shift-left: w294 -> [w298]
                  tunnel: w295 -> [w296] mode=indexing
                  n109 = Enqueue Element(queue=w298, element=w296) -> (queue out=w297:refnum<queue>)  [unwired: 2 in, 2 out]
                }
                n110 = Select(t=TLB_MHL_States."Reset" ("Enum"), s=w289, f=TLB_MHL_States."Task 3" ("Enum")) -> (s? t:f=w290:T5)
              }
              frame 9 {
                n111 = case shown="True" w301 {
                  tunnel: [string[] ["Forward", "Ultrasonic read", "Motor Control"] string[] ["Stop", "Hardware reset", "Software reset", "Motor Control"]] -> w302
                  frame False {
                  }
                  frame True {
                  }
                }
                n112 = for {
                  shift-right: [w311] -> w304
                  shift-left: w303 -> [w312]
                  tunnel: w302 -> [w310] mode=indexing
                  n113 = Enqueue Element(queue=w312, element=w310) -> (queue out=w311:refnum<queue>)  [unwired: 2 in, 2 out]
                }
                n114 = Select(t=TLB_MHL_States."Task 4a" ("Enum"), s=w301, f=TLB_MHL_States."Task 4" ("Enum")) -> (s? t:f=w307:T5)
              }
              frame 10 {
                n115 = Greater Or Equal?(x=w313, y=0.5) -> (x >= y?=w315:bool)
                n116 = case shown="True" w315 {
                  tunnel: [string[] ["Right", "Motor Control"] string[] ["Stop", "Hardware reset", "Software reset", "Motor Control"]] -> w318
                  frame False {
                  }
                  frame True {
                  }
                }
                n117 = for {
                  shift-right: [w325] -> w316
                  shift-left: w317 -> [w326]
                  tunnel: w318 -> [w324] mode=indexing
                  n118 = Enqueue Element(queue=w326, element=w324) -> (queue out=w325:refnum<queue>)  [unwired: 2 in, 2 out]
                }
                n119 = Select(t=TLB_MHL_States."Task 4b" ("Enum"), s=w315, f=TLB_MHL_States."Task 4a" ("Enum")) -> (s? t:f=w319:T5)
              }
              frame 11 {
                n120 = Greater Or Equal?(x=w327, y=0.75) -> (x >= y?=w328:bool)
                n121 = case shown="False" w328 {
                  tunnel: [string[] ["Forward", "Motor control"] string[] ["Stop", "Hardware reset", "Software reset"]] -> w333
                  frame False {
                  }
                  frame True {
                  }
                }
                n122 = for {
                  shift-right: [w339] -> w331
                  shift-left: w332 -> [w340]
                  tunnel: w333 -> [w338] mode=indexing
                  n123 = Enqueue Element(queue=w340, element=w338) -> (queue out=w339:refnum<queue>)  [unwired: 2 in, 2 out]
                }
                n124 = Select(t=TLB_MHL_States."Task 4c" ("Enum"), s=w328, f=TLB_MHL_States."Task 4b" ("Enum")) -> (s? t:f=w330:T5)
              }
              frame 12 {
                n125 = Less Or Equal?(x=w341, y=-0.65) -> (x <= y?=w342:bool)
                n126 = case shown="False" w342 {
                  tunnel: [string[] ["Left", "Motor Control"] string[] ["Stop", "Hardware reset", "Software reset", "Motor Control"]] -> w347
                  frame False {
                  }
                  frame True {
                  }
                }
                n127 = for {
                  shift-right: [w353] -> w344
                  shift-left: w345 -> [w354]
                  tunnel: w347 -> [w352] mode=indexing
                  n128 = Enqueue Element(queue=w354, element=w352) -> (queue out=w353:refnum<queue>)  [unwired: 2 in, 2 out]
                }
                n129 = Select(t=TLB_MHL_States."Task 4d" ("Enum"), s=w342, f=TLB_MHL_States."Task 4c" ("Enum")) -> (s? t:f=w346:T5)
              }
              frame 13 {
                n130 = Or(x=w357, y=w356) -> (x .or. y?=w355:bool)
                n131 = case shown="True" w355 {
                  tunnel: [string[] ["Forward", "Ultrasonic Read", "Motor Control"] string[] ["Stop", "Hardware reset", "Software reset", "Motor Control"]] -> w361
                  frame False {
                  }
                  frame True {
                  }
                }
                n132 = for {
                  shift-right: [w367] -> w359
                  shift-left: w360 -> [w368]
                  tunnel: w361 -> [w366] mode=indexing
                  n133 = Enqueue Element(queue=w368, element=w366) -> (queue out=w367:refnum<queue>)  [unwired: 2 in, 2 out]
                }
                n134 = Select(t=TLB_MHL_States."Startup" ("Enum"), s=w355, f=TLB_MHL_States."Task 4d" ("Enum")) -> (s? t:f=w358:T5)
              }
              frame 5 {
                n135 = for {
                  shift-right: [w374] -> w369
                  shift-left: w370 -> [w375]
                  tunnel: string[] ["Software reset", "Hardware reset", "Motor Control"] -> [w373] mode=indexing
                  n136 = Enqueue Element(queue=w375, element=w373) -> (queue out=w374:refnum<queue>)  [unwired: 2 in, 2 out]
                }
              }
              frame 19 {
                n137 = case shown="False" w376 {
                  tunnel: [string[] ["IR Sensor Read", "Calculate", "Forward", "Motor Control"] string[] ["Hardware reset", "Software reset", "Motor Control"]] -> w377
                  frame False {
                  }
                  frame True {
                  }
                }
                n138 = for {
                  shift-right: [w386] -> w379
                  shift-left: w378 -> [w387]
                  tunnel: w377 -> [w385] mode=indexing
                  n139 = Enqueue Element(queue=w387, element=w385) -> (queue out=w386:refnum<queue>)  [unwired: 2 in, 2 out]
                }
                n140 = Select(t=TLB_MHL_States."Idle" ("Enum"), s=w376, f=TLB_MHL_States."Wall follow mode" ("Enum")) -> (s? t:f=w381:T5)
              }
              frame 20 {
                n141 = Boolean To (0,1)(Boolean=w392) -> (0, 1=w391:i16)
                n142 = Boolean To (0,1)(Boolean=w389) -> (0, 1=w390:i16)
                n143 = formula code="if (stop == 1)\nout = 1;\n\nelse if (detect == 1)\nout = 2;\n\nelse \nout = 0;"("stop"=w391, "detect"=w390) -> ("out"=w393:dbl)
                n144 = case shown="0, Default" w393 {
                  tunnel: [string[] ["Ultrasonic read", "Forward", "NavX Calibrate", "Motor Control"] string[] ["Hardware reset", "Software reset", "Motor Control"] string[] ["Stop", "Motor Control", "Ultrasonic read"]] -> w388
                  frame 0, Default {
                  }
                  frame 1 {
                  }
                  frame 2 {
                  }
                }
                n145 = for {
                  shift-right: [w403] -> w395
                  shift-left: w394 -> [w404]
                  tunnel: w388 -> [w402] mode=indexing
                  n146 = Enqueue Element(queue=w404, element=w402) -> (queue out=w403:refnum<queue>)  [unwired: 2 in, 2 out]
                }
                n147 = Select(t=TLB_MHL_States."Idle" ("Enum"), s=w392, f=TLB_MHL_States."Drive Straight" ("Enum")) -> (s? t:f=w396:u16)
              }
              frame 18 {
                n148 = case shown="True" w405 {
                  tunnel: [string[] ["Cam Acq"] string[] ["Hardware reset", "Software reset", "Cam Exit", ""]] -> w409
                  frame False {
                  }
                  frame True {
                  }
                }
                n149 = for {
                  shift-right: [w415] -> w407
                  shift-left: w408 -> [w416]
                  tunnel: w409 -> [w414] mode=indexing
                  n150 = Enqueue Element(queue=w416, element=w414) -> (queue out=w415:refnum<queue>)  [unwired: 2 in, 2 out]
                }
                n151 = Select(t=TLB_MHL_States."Idle" ("Enum"), s=w405, f=TLB_MHL_States."Acquire image" ("Enum")) -> (s? t:f=w406:T5)
              }
              frame 3 {
              }
              frame 4 {
                # ">>State Logic >>"
                n152 = for {
                  shift-right: [w424] -> w419
                  shift-left: w420 -> [w425]
                  tunnel: string[] ["Software reset", "Hardware reset", "Motor Control", "Cam Exit", "Pre-Exit", "Exit"] -> [w423] mode=indexing
                  n153 = Enqueue Element(queue=w425, element=w423) -> (queue out=w424:refnum<queue>)  [unwired: 2 in, 2 out]
                }
              }
              frame 0 {
              }
            }
          }
        }
        "Main Loop" <- w134
      }
      n154 = while {
        tunnel: w36 -> [w619]
        tunnel: [w618] -> w35
        tunnel: w22 -> [w616]
        tunnel: [w615] -> w34
        tunnel: w28 -> [w614]
        tunnel: [w613] -> w25
        i -> [w612]
        stop <- w617 stop-if-true
        # "EVENT Handling Loop"
        n155 = event shown="[1] <Start Task>: User Event" {
          selector: w619 -> [_ _ _]
          dyn-events: [_ _ _] -> w618
          timeout: _ -> [_ _ _]
          tunnel: [FALSE FALSE w646] -> w617
          tunnel: w616 -> [w624 w631 w644]
          tunnel: [w623 w630 w645] -> w615
          tunnel: w614 -> [w621 w627 w642]
          tunnel: [w620 w626 w641] -> w613
          event Timeout {
            n156 = event-data() -> ()  [unwired: 1 in, 3 out]
            n157 = Enqueue Element(queue=w624, element=TLB_event_states."Idle" ("Enum"), error in (no error)=w621) -> (queue out=w623:refnum<queue>, error out=w620:errorcluster)  [unwired: 1 in, 1 out]
          }
          event User Event {
            n158 = event-data() -> ()  [unwired: 1 in, 5 out]
            n159 = case shown="\"Drive straight\"" "Tasks Selector" {
              tunnel: [TLB_event_states."Idle" ("Enum") TLB_event_states."Start Task 1" ("Enum") TLB_event_states."Start Task 2" ("Enum") TLB_event_states."Start Task 3" ("Enum") TLB_event_states."Start Task 4" ("Enum") TLB_event_states."Wall follow mode" ("Enum") TLB_event_states."Camera vision" ("Enum") TLB_event_states."Start Drive Straight" ("Enum")] -> w628
              frame Default {
              }
              frame "Task 1" {
              }
              frame "Task 2" {
              }
              frame "Task 3" {
              }
              frame "Task 4" {
              }
              frame "Wall following" {
              }
              frame "RT Camera tracking" {
              }
              frame "Drive straight" {
              }
            }
            n160 = Enqueue Element(queue=w631, element=w628, error in (no error)=w627) -> (queue out=w630:refnum<queue>, error out=w626:errorcluster)  [unwired: 1 in, 1 out]
          }
          event User Event {
            n161 = event-data() -> ("Stop Queue"=w646:bool)  [unwired: 1 in, 4 out]
            n162 = Enqueue Element At Opposite End(queue=w644, element=TLB_event_states."Exit" ("Enum"), error in (no error)=w642) -> (queue out=w645:refnum<queue>, error out=w641:errorcluster)  [unwired: 1 in, 1 out]
          }
        }
        "Event handling loop" <- w612
      }
      n163 = while {
        tunnel: w37 -> [w659]
        tunnel: w38 -> [w658]
        tunnel: [w657] -> w44
        tunnel: [w656] -> w43
        tunnel: w42 -> [w655]
        tunnel: [w654] -> w40
        tunnel: w41 -> [w653]
        tunnel: [w652] -> w39
        i -> [w649]
        stop <- w650 stop-if-true
        # "Generate USER Event Loop"
        n164 = local read "DIO 0"() -> (w648:bool)
        n165 = case shown="True" w648 {
          selector: w648 -> [_ w671]
          tunnel: w659 -> [w670 w675]
          tunnel: [w670 w674] -> w656
          tunnel: w655 -> [w669 w673]
          tunnel: [w669 w672] -> w654
          frame False {
          }
          frame True {
            n166 = Generate User Event(user event=w675, event data cluster=w671, error in=w673) -> (user event out=w674:refnum<user-event>, error out=w672:errorcluster)  [unwired: 1 in]
          }
        }
        n167 = case shown="False" "STOP" {
          selector: "STOP" -> [_ w664]
          tunnel: w658 -> [w663 w668]
          tunnel: [w663 w667] -> w657
          tunnel: w653 -> [w662 w666]
          tunnel: [w662 w665] -> w652
          tunnel: [FALSE w664] -> w650
          frame False {
          }
          frame True {
            n168 = Generate User Event(user event=w668, event data cluster=w664, error in=w666) -> (user event out=w667:refnum<user-event>, error out=w665:errorcluster)  [unwired: 1 in]
          }
        }
        n169 = call "FGV Stop.vi"("Init/Read/Write State"=States_for_Action_Engine."Write", "Input Node"=w650) -> ()  [unwired: 1 in, 2 out]
        n170 = Wait (ms)(milliseconds to wait=u32 20) -> ()  [unwired: 1 out]
        "User event loop" <- w649
      }
      n171 = while {
        i -> [w101]
        stop <- w112 stop-if-true
        w102 = 50 ("sample length")
        w117 = T24 [enum."A/AI0"] items=["Not Connected", "AudioIn/Left", "AudioIn/Right", "C/AI0", "C/AI1", "A/AI0", "A/AI1", "A/AI2", "A/AI3", "A/AI4", "A/AI5", "A/AI6", "A/AI7", "B/AI0", "B/AI1", "B/AI2", "B/AI3", "B/AI4", "B/AI5", "B/AI6", "B/AI7", "AI/AI0", "AI/AI1", "AI/AI2", "AI/AI3", "A/AI0 (DIFF)", "A/AI1 (DIFF)", "A/AI2 (DIFF)", "A/AI3 (DIFF)", "B/AI0 (DIFF)", "B/AI1 (DIFF)", "B/AI2 (DIFF)", "B/AI3 (DIFF)"] ("AI Channel")
        w118 = T24 [enum."B/AI0"] items=["Not Connected", "AudioIn/Left", "AudioIn/Right", "C/AI0", "C/AI1", "A/AI0", "A/AI1", "A/AI2", "A/AI3", "A/AI4", "A/AI5", "A/AI6", "A/AI7", "B/AI0", "B/AI1", "B/AI2", "B/AI3", "B/AI4", "B/AI5", "B/AI6", "B/AI7", "AI/AI0", "AI/AI1", "AI/AI2", "AI/AI3", "A/AI0 (DIFF)", "A/AI1 (DIFF)", "A/AI2 (DIFF)", "A/AI3 (DIFF)", "B/AI0 (DIFF)", "B/AI1 (DIFF)", "B/AI2 (DIFF)", "B/AI3 (DIFF)"] ("AI Channel")
        # "IR + Ultrasonic Sensor Loop"
        n172 = call <vilib>:"Ping.vi"("Mxp Side"=Mxp_Selection."MXP B") -> ("CM"=w106:fxp<+,64,16>)  [unwired: 8 in, 2 out]
        "Right Ultrasonic" <- w106
        n173 = call <vilib>:"Ping.vi"("Mxp Side"=Mxp_Selection."MXP A") -> ("CM"=w107:fxp<+,64,16>)  [unwired: 8 in, 2 out]
        "Left Ultrasonic" <- w107
        n174 = call <vilib>:"Sharp IR.vi"("AI Channel"=w118) -> ("Sharp IR Distance"=→"Right IR Sensor":dbl)  [unwired: 8 in, 2 out]
        n175 = call <vilib>:"Sharp IR.vi"("AI Channel"=w117) -> ("Sharp IR Distance"=→"Left IR Sensor":dbl)  [unwired: 8 in, 2 out]
        n176 = Add(x=w107, y=w106) -> (x+y=w109:fxp<+,64,17>)
        n177 = Divide(x=w109, y=fxp<+,64,17> 2.0) -> (x/y=w105:fxp<+,64,64>)
        n178 = call "FGV Stop.vi"("Init/Read/Write State"=States_for_Action_Engine."Read") -> ("Output node"=w112:bool)  [unwired: 2 in, 1 out]
        n179 = call <vilib>:"Median PtByPt.vi"("sample length"=w102, "x"=w105) -> ("median"=w104:dbl)  [unwired: 2 in, 1 out]
        n180 = call <vilib>:"Mode PtByPt.vi"("sample length"=w102, "intervals"=50, "x"=w104) -> ("mode"=→"L/R average" →"Waveform Chart":dbl)  [unwired: 1 in, 1 out]
        n181 = Wait Until Next ms Multiple(millisecond multiple=u32 20) -> ()  [unwired: 1 out]
        "Sensor Loop" <- w101
      }
      n182 = while {
        tunnel: [w92] -> w18
        i -> [w84]
        stop <- w94 stop-if-true
        # "NavX Loop"
        n183 = call <vilib>:"NavX Open.vi"("I2C Channel"=I2C_Channel."A") -> ("NavX Info"=w85:T7)  [unwired: 9 in, 1 out]
        n184 = case shown="True" "NavX Zero Yaw" {
          tunnel: w85 -> [w96 w98]
          tunnel: [w96 w97] -> _
          frame False {
          }
          frame True {
            n185 = call <vilib>:"Zero Yaw.vi"("NavX Info In"=w98) -> ("NavX Info Out"=w97:T7)  [unwired: 10 in]
          }
        }
        n186 = call <vilib>:"YRPHfH.vi"("NavX Info In"=w85) -> ("YRPHfH"=w88:T10)  [unwired: 3 in, 1 out]
        "YRPHfH" <- w88
        n187 = call <vilib>:"Raw Values.vi"("NavX Info In"=w85) -> ("NavX Info Out"=w92:T7)  [unwired: 8 in, 1 out]
        "NavX Info Out" <- w92
        n188 = call <vilib>:"LinearAcceleration.vi"("NavX Info In"=w85) -> ("LinearAcceleration"=→"LinearAcceleration":T8)  [unwired: 9 in, 1 out]
        n189 = call <vilib>:"Displacement.vi"("NavX Info In"=w85) -> ("Displacement"=→"Displacement":T9)  [unwired: 9 in, 1 out]
        n190 = Unbundle By Name(w88) -> ("Yaw"=→"Yaw":dbl)
        n191 = call "FGV Stop.vi"("Init/Read/Write State"=States_for_Action_Engine."Read") -> ("Output node"=w94:bool)  [unwired: 2 in, 1 out]
        n192 = Wait Until Next ms Multiple(millisecond multiple=u32 10) -> ()  [unwired: 1 out]
        "NavX Loop" <- w84
      }
      n193 = while {
        tunnel: w16 -> [w66]
        tunnel: [w65] -> w15
        tunnel: w12 -> [w64]
        tunnel: [w63] -> w11
        tunnel: w10 -> [w62]
        tunnel: [w61] -> w9
        tunnel: w8 -> [w60]
        tunnel: [w59] -> w7
        i -> [w71]
        stop <- w81 stop-if-true
        # "Blackhawk interfacing"
        n194 = call <vilib>:"Blackhawk i2c Open.vi"("I2C Channel"=I2C_Channel."B") -> ("I2C Ref Out"=w55:T26, "error out"=w54:errorcluster)  [unwired: 2 in]
        n195 = call <vilib>:"Blackhawk DIO Read.vi"("I2C Ref In"=w55, "PIN"=u8 0, "error in (no error)"=w54) -> ("I2C Ref Out"=w79:T26, "error out"=w80:errorcluster)  [unwired: 3 in, 1 out]
        n196 = call <vilib>:"C DIO Read.vi"("error in (no error)"=w60, "DIO Info In in"=w64) -> ("error out"=w59:errorcluster, "IN"=→"DIO 1":bool, "DIO Info In out"=w63:T21)  [unwired: 7 in]
        n197 = call <vilib>:"C DIO Read.vi"("error in (no error)"=w62, "DIO Info In in"=w66) -> ("error out"=w61:errorcluster, "IN"=→"DIO 0":bool, "DIO Info In out"=w65:T21)  [unwired: 7 in]
        n198 = call <vilib>:"Blackhawk Relay.vi"("error in (no error)"=w80, "On/Off"="On/Off", "Relay"=enum8{"Relay 0", "Relay 1", "Relay 2"}."Relay 0", "I2C Ref In"=w79) -> ("error out"=w76:errorcluster, "I2C Ref Out"=w73:T26)  [unwired: 6 in]
        n199 = call <vilib>:"Blackhawk Servo.vi"("error in (no error)"=w76, "Servo Select"=enum16{"Servo 5", "Servo 6"}."Servo 5", "Servo Angle"="Servo Angle", "I2C Ref In"=w73) -> ("error out"=w70:errorcluster, "I2C Ref Out"=w69:T26)  [unwired: 6 in]
        n200 = call <vilib>:"RT Get CPU Loads.vi"() -> ("error out"=→"Load":errorcluster, "CPU loads"=→"CPU loads":T1[])  [unwired: 10 in]
        n201 = call <vilib>:"Blackhawk read Limit.vi"("error in (no error)"=w70, "I2C Ref In"=w69) -> ("error out"=→"Blackhawk error":errorcluster, "Limit Switch Array"=→"Limit Switch Array":bool[])  [unwired: 1 in, 1 out]
        n202 = call "FGV Stop.vi"("Init/Read/Write State"=States_for_Action_Engine."Read") -> ("Output node"=w81:bool)  [unwired: 2 in, 1 out]
        n203 = Wait (ms)(milliseconds to wait=u32 20) -> ()  [unwired: 1 out]
        "Blackhawk loop" <- w71
      }
      n204 = while {
        tunnel: w23 -> [w128]
        tunnel: w22 -> [w125]
        i -> [w119]
        stop <- w122 stop-if-true
        # "Status Loop for Action Queues"
        n205 = Get Queue Status(queue=w128, return elements? (F)=TRUE) -> (error out=w124:errorcluster, # elements in queue=→"Action Queue Items":i32, elements=→"Action Queues items":string[])  [unwired: 1 in, 5 out]
        n206 = Get Queue Status(queue=w125, return elements? (F)=TRUE) -> (# pending remove=→"State Logic Queue Items":i32, error out=w123:errorcluster)  [unwired: 1 in, 6 out]
        n207 = Merge Errors(w124, w123) -> (w122:errorcluster)
        n208 = Wait (ms)(milliseconds to wait=u32 500) -> ()  [unwired: 1 out]
        "Status loop" <- w119
      }
      n209 = call <vilib>:"DIO Close.vi"("error in (no error)"=w9, "DIO Info In"=w15) -> ()  [unwired: 9 in, 1 out]
      n210 = call <vilib>:"DIO Close.vi"("error in (no error)"=w7, "DIO Info In"=w11) -> ()  [unwired: 9 in, 1 out]
      n211 = while {
        stop <- w49 stop-if-true
        # "Motor Control Loop"
        n212 = Wait Until Next ms Multiple(millisecond multiple=u32 5) -> ()  [unwired: 1 out]
        n213 = call "New motor Control integrated remodeled.vi"("States"=enum16{"RESET ENCODER", "WRITE", "READ", "INIT"}."READ") -> ("Speed and distance cluster"=→"Speed and distance cluster":T2)  [unwired: 4 in, 1 out]
        n214 = call "FGV Stop.vi"("Init/Read/Write State"=States_for_Action_Engine."Read") -> ("Output node"=w49:bool)  [unwired: 2 in, 1 out]
      }
      n215 = call <vilib>:"NavX Close.vi"("NavX Info In"=w18) -> ()  [unwired: 10 in, 1 out]
      n216 = Merge Errors "Merge Errors"(w40, w39) -> (w21:errorcluster)
      n217 = Merge Errors(w25, w21) -> (w4:errorcluster)
      n218 = Destroy User Event(user event=w43, error in=w4) -> ()  [unwired: 1 out]
      n219 = Destroy User Event(user event=w44, error in=w4) -> ()  [unwired: 1 out]
      n220 = Unregister For Events(event registration refnum=w35, error in=w4) -> ()  [unwired: 1 out]
      n221 = Release Queue(queue=w6, error in (no error)=w4) -> (error out=→"error out":errorcluster)  [unwired: 1 in, 2 out]
      n222 = Release Queue(queue=w34, error in (no error)=w4) -> ()  [unwired: 1 in, 3 out]
    }
    frame #2 {
      n223 = call "New motor Control integrated remodeled.vi"("States"=enum16{"RESET ENCODER", "WRITE", "READ", "INIT"}."WRITE", "Target Speed"=T20 {"xTargetSpeed"=0.0, "yTargetSpeed"=0.0, "wTargetSpeed"=0.0}) -> ()  [unwired: 3 in, 2 out]
    }
    frame #3 {
    }
  }
